vi "quad11.vi"() -> ()   [LabVIEW 2010]
uses:
  <vilib>/measure/matone.llb/Extract Single Tone Information 1 Chan.vi
  <vilib>/measure/NI_MAPro.lvlib
panel:
  in  "Tab Control":enum32{"Page 1", "Page 2"}(tab)
  out "XY Graph":cluster{sgl[], "q":i32[]}(graph)
  out "Intensity Graph":dbl[][](graph)
  out "detected phase (deg)":dbl format="%#_4p"
  out "detected frequency":dbl format="%.2p"
  out "i":i32
  out "zero":dbl[](array[numeric])
  out "quad":dbl[](array[numeric])
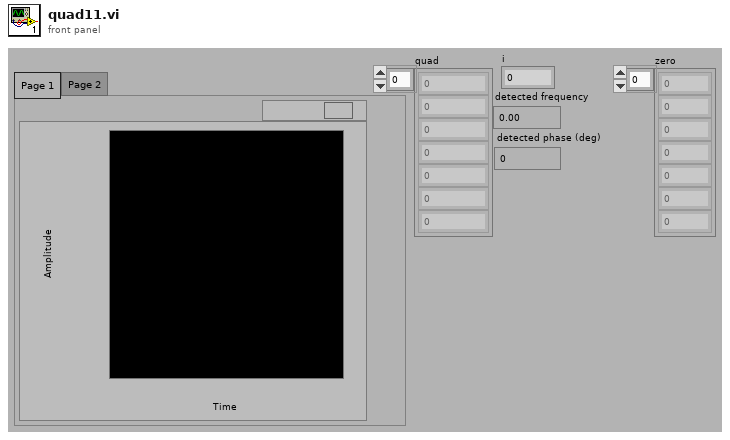
[diagram p1: front panel]
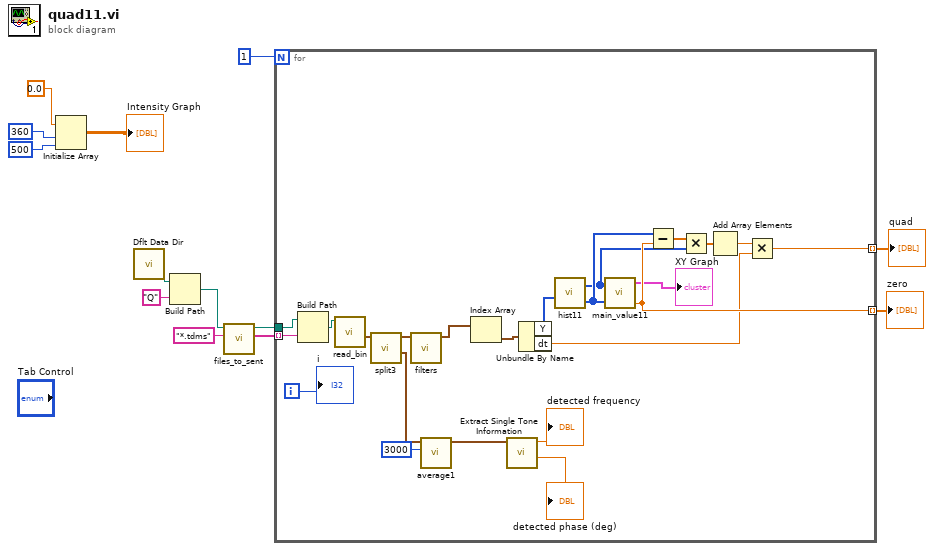
[diagram p0: block diagram]
diagram:
  n1 = Initialize Array(0.0 ("element"), 360 ("dimension size"), 500 ("dimension size")) -> (→"Intensity Graph":dbl[][])
  n2 = call <vilib>:"Dflt Data Dir.vi"() -> ("App:Default Data Directory"=w10:path)
  n3 = Build Path(base path=w10, name or relative path="Q") -> (appended path=w8:path)
  n4 = call "files_to_sent.vi"("pattern"="*.tdms", "Directory"=w8) -> ("names"=w12:string[], "directory dup"=w11:path)  [unwired: 2 in, 2 out]
  n5 = for {
    N: 1 -> [_]
    tunnel: w12 -> [w34] mode=indexing
    tunnel: w11 -> [w35]
    tunnel: [w31] -> w1 mode=indexing
    tunnel: [w30] -> w2 mode=indexing
    i -> [w29]
    n6 = Build Path(base path=w35, name or relative path=w34) -> (appended path=w36:path)
    n7 = call "read_bin.vi"("datalog path"=w36) -> ("Waveform Graph"=w33:waveform(i16)[])  [unwired: 3 in, 3 out]
    n8 = call "split3.vi"("Array of Waveform In"=w33) -> ("Sync"=w28:waveform(i16), "Array of Waveform"=w32:waveform(i16)[])  [unwired: 5 in]
    n9 = call "filters.vi"("Array"=w32) -> ("Array 2"=w23:waveform(i16)[])  [unwired: 6 in]
    n10 = call "average1.vi"("Size"=3000, "SignalIn"=w28) -> ("output waveform"=w27:waveform(i16))  [unwired: 5 in]
    n11 = Index Array(array=w23) -> (element=w22:waveform(i16))  [unwired: 1 in]
    n12 = call-poly <vilib>:"Extract Single Tone Information.vi"("time signal in"=w27) -> ("detected phase (deg)"=→"detected phase (deg)":dbl, "detected frequency"=→"detected frequency":dbl)  [unwired: 5 in, 4 out]
    n13 = Unbundle By Name(w22) -> ("Y"=w21:i16[], "dt"=w15:dbl)
    n14 = call "hist11.vi"("Y"=w21) -> ("values"=w18:i16[], "q"=w16:i32[])  [unwired: 3 in]
    n15 = call "main_value11.vi"("values"=w18, "q"=w16) -> ("main"=w31:dbl, "hist"=→"XY Graph":cluster{sgl[], "q":i32[]})  [unwired: 1 in]
    n16 = Subtract(x=w18, y=w31) -> (x-y=w19:dbl[])
    n17 = Multiply(x=w19, y=w16) -> (x*y=w20:dbl[])
    n18 = Add Array Elements(numeric array=w20) -> (sum=w17:dbl)
    n19 = Multiply(x=w17, y=w15) -> (x*y=w30:dbl)
    "i" <- w29
  }
  "quad" <- w2
  "zero" <- w1
